vi "Find Group Shared Path.vi"(11 "Group Filtered Path map":map{string, string[]}(c390)) -> (3 "Found Common Paths":string[](array[string]))   [LabVIEW 2019, in "Project.Dependencies Finder.lvlib" / "Dependency Source.lvclass"]
doc: "Find common paths that might be used to identify the package."
uses:
  Dependency Source.lvclass
  d34327d4-a2bb-4fe5-866c-5703ea76e9e5.vi
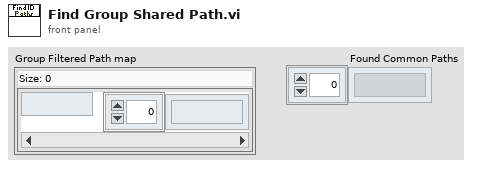
[diagram p1: front panel]
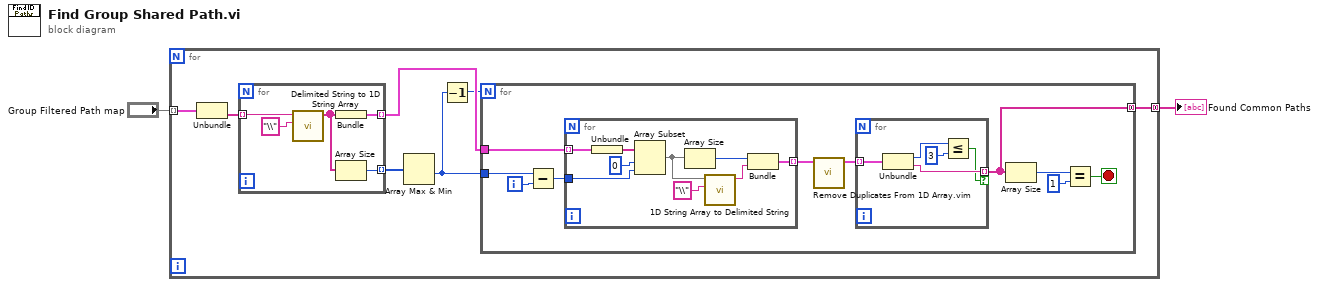
[diagram p0: block diagram]
diagram:
  n1 = for {
    tunnel: "Group Filtered Path map" -> [w9] mode=indexing
    tunnel: [w3] -> w2 mode=concatenating
    n2 = Unbundle(w9) -> ("value"=w8:string[])  [unwired: 1 out]
    n3 = for {
      tunnel: w8 -> [w37] mode=indexing
      tunnel: [w36] -> w7 mode=indexing
      tunnel: [w34] -> w6 mode=indexing
      n4 = call <vilib>:"Delimited String to 1D String Array.vi"("delimiter"="\\" ("search string"), "delimited string"=w37) -> ("string array"=w35:string[])  [unwired: 9 in]
      n5 = Bundle("string array"=w35) -> (w34:cluster{"string array":string[]})  [unwired: 1 in]
      n6 = Array Size(array=w35) -> (size(s)=w36:i32)
    }
    n7 = Array Max & Min(array=w7) -> (min value=w4:i32)  [unwired: 3 out]
    n8 = Decrement(x=w4) -> (x-1=w5:i32)
    n9 = for {
      N: w5 -> [_]
      tunnel: w6 -> [w19]
      tunnel: w4 -> [w18]
      tunnel: [w10] -> w3 mode=concatenating
      i -> [w17]
      stop <- w14 stop-if-true
      n10 = Subtract(x=w18, y=w17) -> (x-y=w16:i32)
      n11 = for {
        tunnel: w19 -> [w33] mode=indexing
        tunnel: w16 -> [w31]
        tunnel: [w25] -> w12 mode=indexing
        n12 = Unbundle(w33) -> ("string array"=w32:string[])
        n13 = Array Subset(array=w32, index=0, length=w31) -> (w28:string[])
        n14 = Array Size(array=w28) -> (size(s)=w27:i32)
        n15 = call <vilib>:"1D String Array to Delimited String.vi"("delimiter"="\\" ("search string"), "string array"=w28) -> ("delimited string"=w26:string)  [unwired: 9 in]
        n16 = Bundle(w27, "delimited string"=w26) -> (w25:cluster{i32, "delimited string":string})  [unwired: 1 in]
      }
      n17 = call "Remove Duplicates From 1D Array.vim"("array"=w12) -> ("array with duplicates removed"=w11:cluster{i32, "delimited string":string}[])  [unwired: 10 in]
      n18 = for {
        tunnel: w11 -> [w24] mode=indexing
        tunnel: [w21] -> w10 mode=indexing if=w20
        n19 = Unbundle(w24) -> (w23:i32, "delimited string"=w21:string)
        n20 = Less Or Equal?(x=w23, y=3) -> (x <= y?=w20:bool)
      }
      n21 = Array Size(array=w10) -> (size(s)=w13:i32)
      n22 = Equal?(x=w13, y=1) -> (x = y?=w14:bool)
    }
  }
  "Found Common Paths" <- w2
